vi "test Import Acyclic Frames.vi"(8 "error in":errorcluster, 11 "TestCase in":refnum<class "1553 Parameters Import.lvclass">) -> (0 "error out":errorcluster, 3 "TestCase out":refnum<class "1553 Parameters Import.lvclass">)   [LabVIEW 2020, in "1553 Parameters Import.lvclass"]
uses:
  1553 Parameters Import.lvclass
  1553 Parameters Import.lvclass/1553 Parameters Import.ctl
  <vilib>/addons/_JKI Toolkits/VI Tester/TestCase.llb/TestCase.lvclass
  C:/Program Files (x86)/National Instruments/LabVIEW 2020/vi.lib/addons/_JKI Toolkits/VI Tester/TestCase.llb/TestCase.lvclass
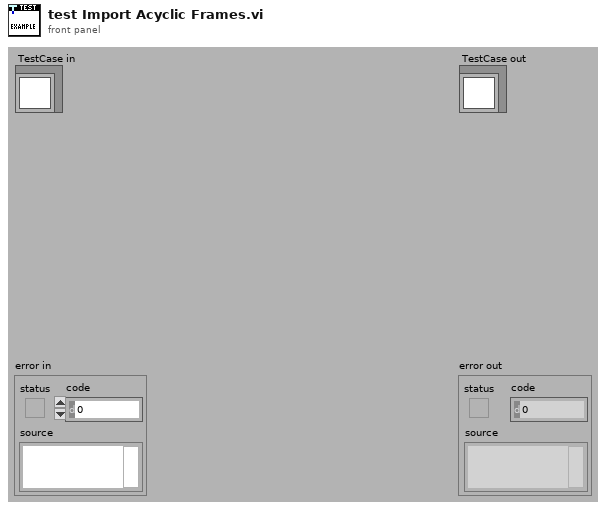
[diagram p1: front panel]
types:
  T1 = typedef "1553 Channel.ctl" = cluster{"HW channel":u16, "terminals":T2[], "messages":T4[], "acyclic frame names":string[]}
  T2 = typedef "Terminal Name and Address.ctl" = cluster{"name":string, "terminal address":T3}
  T3 = typedef "Address.ctl" = u16
  T4 = typedef "Message Definition.ctl" = cluster{"name":string, "message type":T5, "endpoint Rx":T6, "endpoint Tx":T6, "mode code":u16, "number of words":u16, "parameters":cluster{"name":string, "default value":dbl, "unit":string, "parameter definition":T7}[], "create timestamp channel":bool}
  T5 = typedef "Message Type.ctl" = string
  T6 = typedef "Terminal Endpoint.ctl" = cluster{"terminal address":T3, "subaddress":T3}
  T7 = typedef "Parameter Definition.ctl" = cluster{"start index":i32, "size (bits)":i32, "encoding":enum16{"BNR", "BCD", "Discrete"}, "signed":bool, "multiplier":dbl, "offset":dbl}
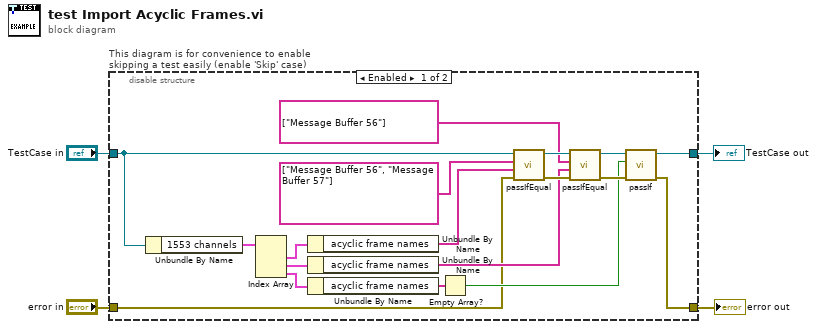
[diagram p0: block diagram]
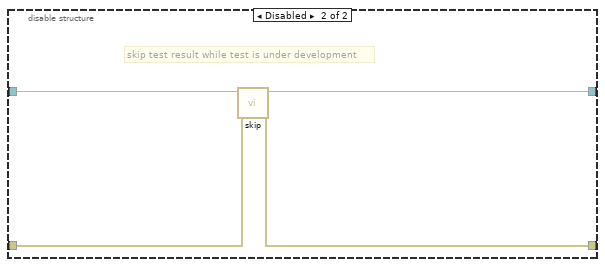
[diagram p2: hidden frame]
diagram:
  n1 = disable-structure "This diagram is for convenience to enable skipping a test easily (enable 'Skip' case)" shown="Enabled" {
    disable-tunnel: "TestCase in" -> [w6 w26]
    disable-tunnel: [w11 w24] -> w1
    disable-tunnel: [w12 w25] -> w3
    disable-tunnel: "error in" -> [w7 w23]
    frame Enabled {
      n2 = Unbundle By Name(w6) -> ("1553 channels"=w5:T1[])
      n3 = Index Array(array=w5) -> (element #1=w22:T1, element #2=w20:T1, element #3=w10:T1)  [unwired: 3 in]
      n4 = Unbundle By Name(w22) -> ("acyclic frame names"=w18:string[])
      n5 = Unbundle By Name(w20) -> ("acyclic frame names"=w15:string[])
      n6 = Unbundle By Name(w10) -> ("acyclic frame names"=w9:string[])
      n7 = Empty Array?(array=w9) -> (empty?=w8:bool)
      n8 = call-dynamic "passIfEqual.vi"("error in (no error)"=w7, "y"=w18, "x"=string[] ["Message Buffer 56", "Message Buffer 57"] ("acyclic frame names"), "TestCase in"=w6) -> ("error out"=w21:errorcluster, "TestCase out"=w19:refnum<class "1553 Parameters Import.lvclass">)  [unwired: 6 in]
      n9 = call-dynamic "passIfEqual.vi"("error in (no error)"=w21, "y"=w15, "x"=string[] ["Message Buffer 56"] ("acyclic frame names"), "TestCase in"=w19) -> ("error out"=w14:errorcluster, "TestCase out"=w13:refnum<class "1553 Parameters Import.lvclass">)  [unwired: 6 in]
      n10 = call-dynamic "passIf.vi"("error in (no error)"=w14, "pass"=w8, "TestCase in"=w13) -> ("error out"=w12:errorcluster, "TestCase out"=w11:refnum<class "1553 Parameters Import.lvclass">)  [unwired: 7 in]
    }
    frame Disabled {
      # "skip test result while test is under development"
      n11 = call <vilib>:"skip.vi"("error in (no error)"=w23, "TestCase in"=w26) -> ("error out"=w25:errorcluster, "TestCase out"=w24:refnum<class "1553 Parameters Import.lvclass">)  [unwired: 8 in]
    }
  }
  "error out" <- w3
  "TestCase out" <- w1
